vi "Pre Launch Init.vi"(11 "FirstAF in":refnum<class "FirstAF.lvclass">) -> (0 "error out":errorcluster, 3 "FirstAF out":refnum<class "FirstAF.lvclass">)   [LabVIEW 2019, in "FirstAF.lvlib" / "FirstAF.lvclass"]
doc: "(<B>Filename</B>: Actor Framework.lvlib:Actor.lvclass:Pre Launch Init.vi)\n\nDefines behavior that occurs after the Launch Nested Actor method is invoked but before the actor's Actor Core method begins running.\n\nBy default, this method does nothing. A descendant class may override it to define behavior."
uses:
  FirstAF.lvclass
  FirstAF.lvclass/FirstAF.ctl
  <vilib>/ActorFramework/Actor/Actor.lvclass
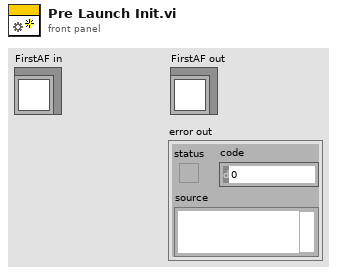
[diagram p1: front panel]
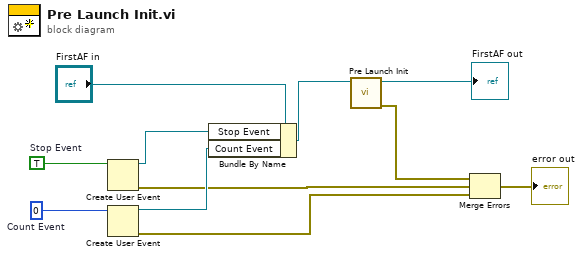
[diagram p0: block diagram]
diagram:
  w11 = 0  # Count Event
  w10 = TRUE  # Stop Event
  n1 = Create User Event(user event datatype=w10) -> (user event=w1:refnum<user-event>, error out=w7:errorcluster)  [unwired: 1 in]
  n2 = Create User Event(user event datatype=w11) -> (user event=w8:refnum<user-event>, error out=w6:errorcluster)  [unwired: 1 in]
  n3 = Bundle By Name(cluster="FirstAF in", "Stop Event"=w1, "Count Event"=w8) -> (w5:refnum<class "FirstAF.lvclass">)
  n4 = call-parent "Pre Launch Init.vi"("Actor in"=w5) -> ("error out"=w3:errorcluster, "Actor out"=→"FirstAF out":refnum<class "FirstAF.lvclass">)  [unwired: 9 in]
  n5 = Merge Errors(w3, w7, w6) -> (→"error out":errorcluster)
